vi "config_model.vi"(8 "error in (no error)":errorcluster) -> (0 "error out":errorcluster)   [LabVIEW 2020, in "lv_documentation.lvlib"]
uses:
  lv_documentation.lvlib
  <vilib>/Utility/config.llb/Write Key (String).vi
  <vilib>/Utility/config.llb/NI_LVConfig.lvlib
  <vilib>/httpClient/LabVIEWHTTPClient.lvlib
panel:
  in  "key":string
  in  "Provider Selector":enum32{"OpenAI", "Gemini"}(tab)
  in  "openai_model_name":string(combo)="gpt-4o-mini" caption="model_name"
  in  "gemini_model_name":string(combo)="gemini-2.0-flash" caption="model_name"
  in  "Configure":bool
  # "Select Provider and Model and Enter API Key"
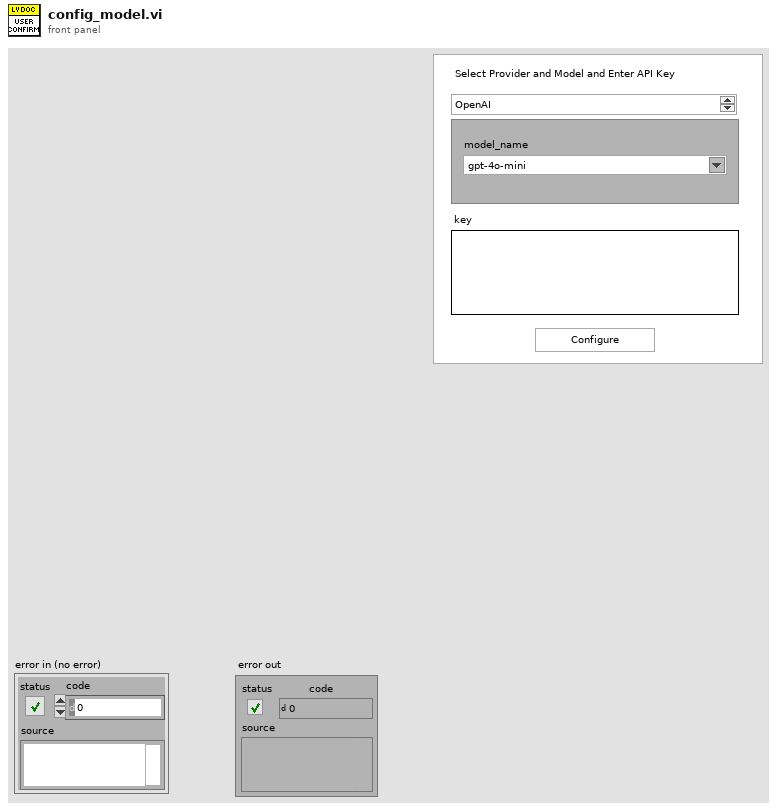
[diagram p1: front panel]
types:
  T1 = typedef "NI_LVConfig.lvlib/Config Data RefNum.ctl" = refnum<k1>
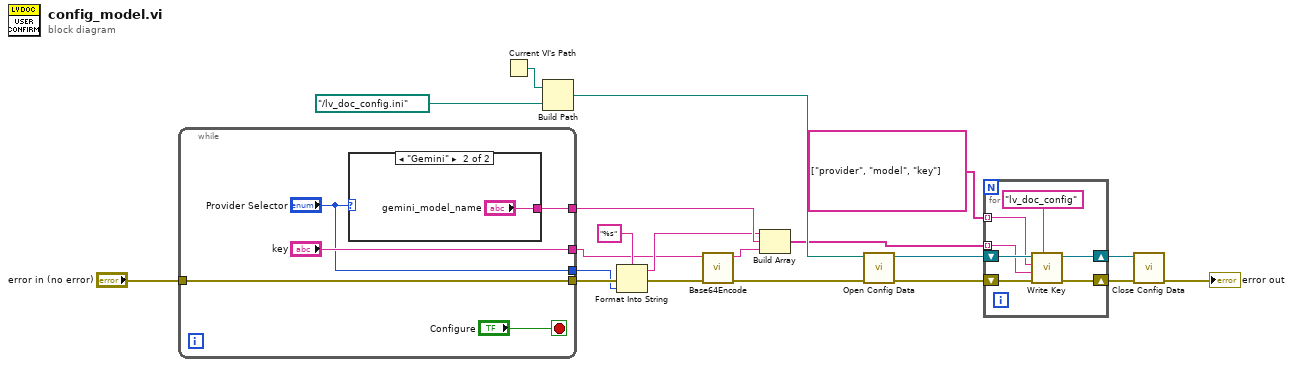
[diagram p0: block diagram]
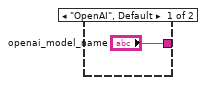
[diagram p2: hidden frame]
diagram:
  n1 = while {
    tunnel: "error in (no error)" -> [w25]
    tunnel: [w25] -> w19
    tunnel: ["key"] -> w4
    tunnel: [w22] -> w10
    tunnel: ["Provider Selector"] -> w8
    stop <- "Configure" stop-if-true
    n2 = case shown="\"Gemini\"" "Provider Selector" {
      tunnel: ["openai_model_name" "gemini_model_name"] -> w22
      frame "OpenAI", Default {
      }
      frame "Gemini" {
      }
    }
  }
  n3 = Current VI's Path() -> (path=w16:path)
  n4 = Build Path(base path=w16, name or relative path=path "../lv_doc_config.ini") -> (appended path=w14:path)
  n5 = Format Into String(format string="%s", error in=w19, w8) -> (resulting string=w7:string, error out=w2:errorcluster)  [unwired: 1 in]
  n6 = call <vilib>:"Base64Encode.vi"("error in (no error)"=w2, "buffer in"=w4) -> ("error out"=w1:errorcluster, "encoded string"=w3:string)  [unwired: 8 in]
  n7 = Build Array(w7, w10, w3) -> (w9:string[])
  n8 = call <vilib>:"Open Config Data.vi"("error in (no error)"=w1, "configuration file path"=w14) -> ("error out"=w18:errorcluster, "refnum"=w12:T1)  [unwired: 7 in, 1 out]
  n9 = for {
    shift-right: [w33] -> w13
    shift-left: w18 -> [w34]
    shift-right: [w31] -> w11
    shift-left: w12 -> [w32]
    tunnel: w9 -> [w29] mode=indexing
    tunnel: string[] ["provider", "model", "key"] ("appended array") -> [w28] mode=indexing
    n10 = call-poly <vilib>:"Write Key.vi"("section"="lv_doc_config", "error in (no error)"=w34, "value"=w29, "key"=w28, "refnum"=w32) -> ("error out"=w33:errorcluster, "refnum out"=w31:T1)  [unwired: 4 in, 1 out]
  }
  n11 = call <vilib>:"Close Config Data.vi"("error in (no error)"=w13, "refnum"=w11) -> ("error out"=→"error out":errorcluster)  [unwired: 8 in, 1 out]
